vi "test-002.vi"() -> ()   [LabVIEW 2019]
uses:
  <vilib>/addons/control/pid/NI_PID_pid.lvlib
  <vilib>/ptbypt/NI_PtbyPt.lvlib
panel:
  out "Waveform Chart":T1(graph)
  in  "J":dbl
  in  "A":dbl
  in  "V":dbl=10.0 format="%#_13g"
  in  "D":dbl=20.0 format="%#_13g"
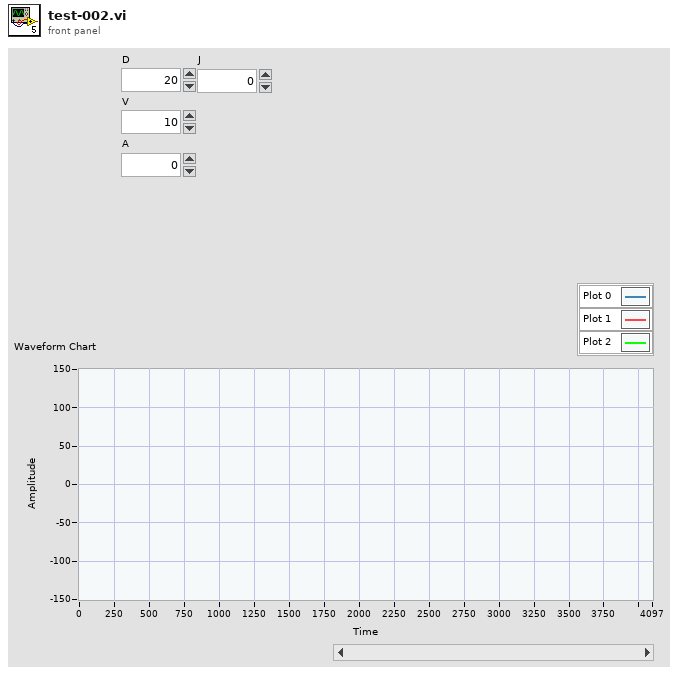
[diagram p1: front panel]
types:
  T1 = cluster{"setpoint":dbl, "integral x(t)":dbl, "integral x(t)":dbl}
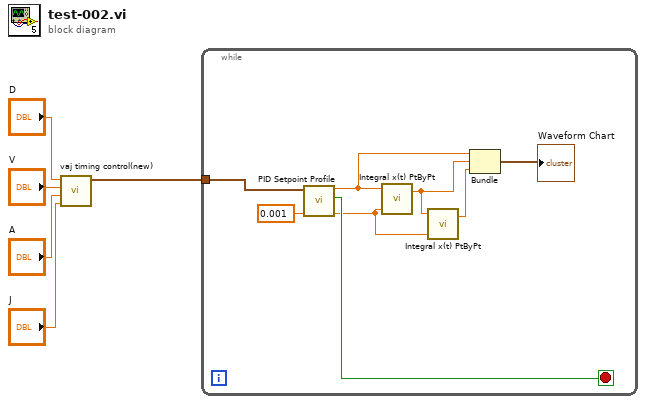
[diagram p0: block diagram]
diagram:
  n1 = call "vaj timing control(new).vi"("J"="J", "A"="A", "V"="V", "D"="D") -> ("Array"=w1:cluster{"Numeric":dbl, "Numeric":dbl}[])  [unwired: 7 in]
  n2 = while {
    tunnel: w1 -> [w13]
    stop <- w11 stop-if-true
    n3 = call <vilib>:"PID Setpoint Profile.vi"("dt (s)"=0.001, "setpoint profile"=w13) -> ("dt out (s)"=w8:dbl, "profile complete?"=w11:bool, "setpoint"=w10:dbl)  [unwired: 4 in, 1 out]
    n4 = call <vilib>:"Integral x(t) PtByPt.vi"("dt"=w8, "x"=w10) -> ("integral x(t)"=w9:dbl)  [unwired: 2 in, 1 out]
    n5 = call <vilib>:"Integral x(t) PtByPt.vi"("dt"=w8, "x"=w9) -> ("integral x(t)"=w7:dbl)  [unwired: 2 in, 1 out]
    n6 = Bundle("setpoint"=w10, "integral x(t)"=w9, "integral x(t)"=w7) -> (→"Waveform Chart":T1)  [unwired: 1 in]
  }
